vi "midi_ParseHeader.vi"(8 "error in (no error)":errorcluster, 11 "string in":string) -> (0 "error out":errorcluster, 2 "header info":T1, 3 "string out":string)   [LabVIEW 2013]
doc: "Read the header chunk of a standard MIDI file."
panel:
  # "midi_ParseHeader"
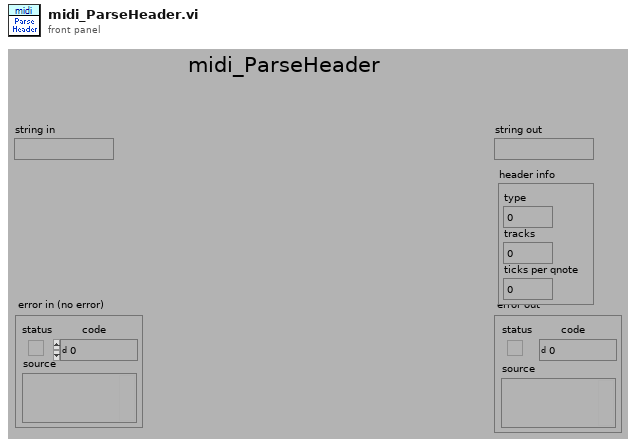
[diagram p1: front panel]
types:
  T1 = cluster{"type":u16, "tracks":u16, "ticks per qnote":u16}
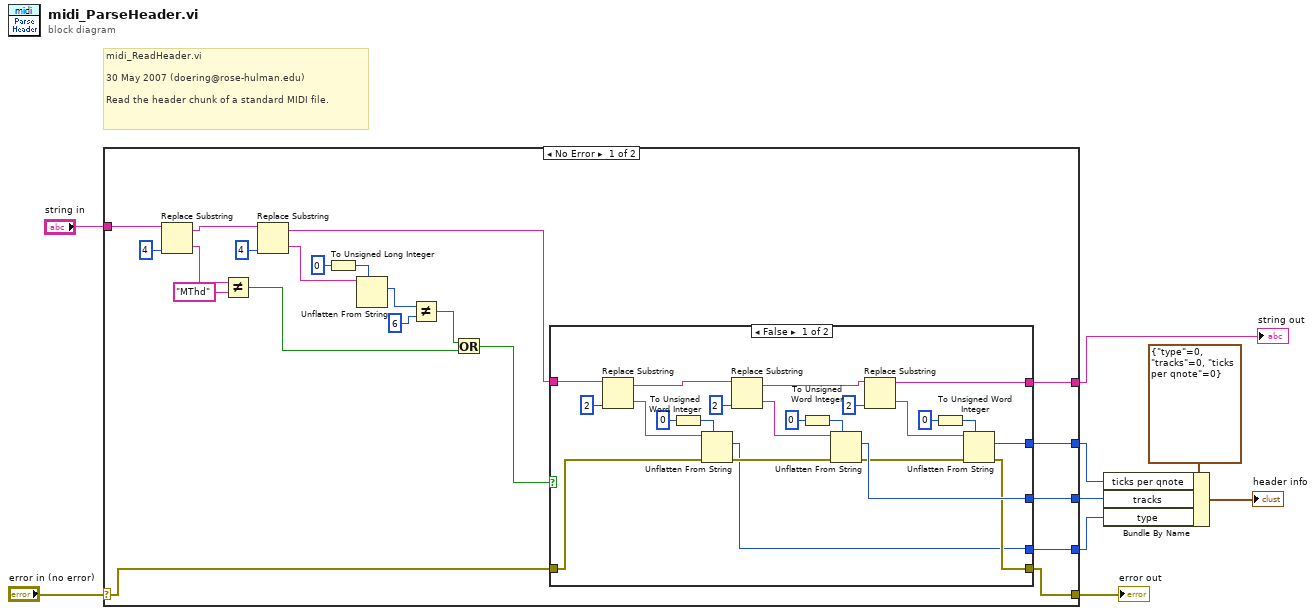
[diagram p0: block diagram]
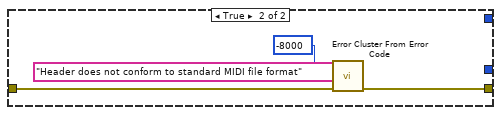
[diagram p2: hidden frame]
diagram:
  # "midi_ReadHeader.vi\n\n30 May 2007 (doering@rose-hulman.edu)\n\nRead the header chunk of a standard MIDI file."
  n1 = case shown="No Error" "error in (no error)" {
    selector: "error in (no error)" -> [w27 w58]
    tunnel: [w15 w58] -> w8
    tunnel: "string in" -> [w30 _]
    tunnel: [w13 _] -> w2
    tunnel: [w12 _] -> w3
    tunnel: [w11 _] -> w4
    tunnel: [w10 _] -> w6
    frame No Error {
      n2 = Replace Substring(2:4 ("length (len. of substring)"), 5:w30) -> (0:w29:string, 1:w24:string)  [unwired: 2 in]
      n3 = Not Equal?(x=w29, y="MThd") -> (x != y?=w17:bool)
      n4 = Replace Substring(2:4 ("length (len. of substring)"), 5:w24) -> (0:w21:string, 1:w14:string)  [unwired: 2 in]
      n5 = To Unsigned Long Integer(number=u32 0) -> (unsigned 32bit integer=w22:u32)
      n6 = Unflatten From String(type=w22, binary string=w21) -> (value=w20:u32)  [unwired: 3 in, 2 out]
      n7 = Not Equal?(x=w20, y=u32 6) -> (x != y?=w18:bool)
      n8 = Or(x=w18, y=w17) -> (x .or. y?=w16:bool)
      n9 = case shown="False" w16 {
        tunnel: w27 -> [w48 w55]
        tunnel: [w33 w54] -> w15
        tunnel: w14 -> [w49 _]
        tunnel: [w31 _] -> w13
        tunnel: [w36 _] -> w12
        tunnel: [w35 _] -> w11
        tunnel: [w32 _] -> w10
        frame False {
          n10 = Replace Substring(2:2 ("length (len. of substring)"), 5:w49) -> (0:w50:string, 1:w44:string)  [unwired: 2 in]
          n11 = To Unsigned Word Integer(number=u32 0) -> (unsigned 16bit integer=w51:u16)
          n12 = Unflatten From String(type=w51, binary string=w50, error in (no error)=w48) -> (value=w31:u16, error out=w42:errorcluster)  [unwired: 2 in, 1 out]
          n13 = Replace Substring(2:2 ("length (len. of substring)"), 5:w44) -> (0:w47:string, 1:w37:string)  [unwired: 2 in]
          n14 = To Unsigned Word Integer(number=u32 0) -> (unsigned 16bit integer=w43:u16)
          n15 = Unflatten From String(type=w43, binary string=w47, error in (no error)=w42) -> (value=w36:u16, error out=w34:errorcluster)  [unwired: 2 in, 1 out]
          n16 = Replace Substring(2:2 ("length (len. of substring)"), 5:w37) -> (0:w38:string, 1:w32:string)  [unwired: 2 in]
          n17 = To Unsigned Word Integer(number=u32 0) -> (unsigned 16bit integer=w41:u16)
          n18 = Unflatten From String(type=w41, binary string=w38, error in (no error)=w34) -> (value=w35:u16, error out=w33:errorcluster)  [unwired: 2 in, 1 out]
        }
        frame True {
          n19 = call <vilib>:"Error Cluster From Error Code.vi"("error in (no error)"=w55, "error message (\"\")"="Header does not conform to standard MIDI file format" ("error message (\"\")"), "error code (0)"=-8000) -> ("error out"=w54:errorcluster)  [unwired: 6 in]
        }
      }
    }
    frame Error {
    }
  }
  "error out" <- w8
  "string out" <- w6
  n20 = Bundle By Name(cluster=T1 {"type"=0, "tracks"=0, "ticks per qnote"=0}, "ticks per qnote"=w4, "tracks"=w3, "type"=w2) -> (→"header info":T1)
